vi "_Write_Query.vi"(8 "error in (no error)":errorcluster, 11 "Postgres Connector In":refnum<class "Postgres Connector.lvclass">) -> (0 "error out":errorcluster)   [LabVIEW 2019, in "PG_LIB.lvlib" / "Postgres Connector.lvclass"]
doc: "This VI is used to send a command to the PostgreSQL database"
uses:
  Postgres Connector.lvclass
  Postgres Connector.lvclass/Postgres Connector.ctl
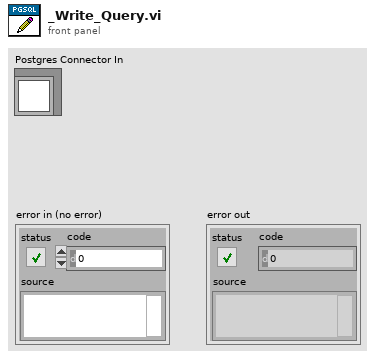
[diagram p1: front panel]
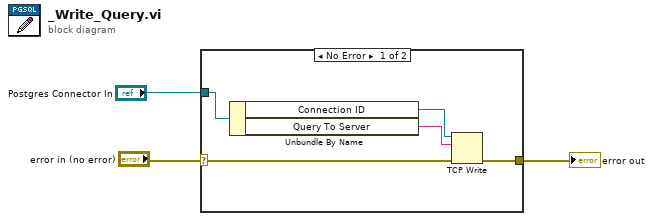
[diagram p0: block diagram]
diagram:
  n1 = case shown="No Error" "error in (no error)" {
    selector: "error in (no error)" -> [w7 w9]
    tunnel: "Postgres Connector In" -> [w6 _]
    tunnel: [w5 w9] -> w1
    frame No Error {
      n2 = Unbundle By Name(w6) -> ("Connection ID"=w8:refnum<k5>, "Query To Server"=w4:string)
      n3 = TCP Write(connection ID=w8, data in=w4, error in (no error)=w7) -> (error out=w5:errorcluster)  [unwired: 1 in, 2 out]
    }
    frame Error {
    }
  }
  "error out" <- w1
